vi "Teststand Edit STP Sent Command.vi"(8 "error in":errorcluster, 10 "STP Set Profile Data in":T1={"ECU CAN Port"="CAN1", "CMD"=133, "CAN Write Data"=[], "+veResponseCode"=160} {"+veResponseCode" format="%.0x"; "CMD" items=["TSW_VERSION(130)"=130, "WAIT_EVENT(132)"=132, "SEQUENCER(133)"=133, "TSW_RESET(150)"=150, "CONFIG_ECU(151)"=151, "TEST_CORE (152)"=152, "TEST_WATCHDOG (153)"=153, "TEST_MONITORING (154)"=154, "READ_MEMORY (162)"=162, "WRITE_ERASE_MEMORY (164)"=164, "COMM_EXTERNAL (190)"=190, "COMM_INTERNAL (195)"=195, "GET_ANALOG_INPUT (210)"=210, "GET_DIGITAL_INPUT (211)"=211, "GET_FREQUENCY_INPUT (212)"=212, "TEST_INPUT_STRUCTURE (214)"=214, "GENERATE_OUTPUT_SIGNAL (220)"=220, "GENERATE_SYNCHRONIZED_OUTPUT_SIGNALS (221)"=221, "eDCU_Specific (250)"=250]; "CAN Write Data" format="%.0x"}, 11 "Sequence Context In":refnum<k7>) -> (0 "error out":errorcluster, 3 "STP Profile Data Out":T1={"ECU CAN Port"="CAN1", "CMD"=133, "CAN Write Data"=[], "+veResponseCode"=160} {"+veResponseCode" format="%.0x"; "CMD" items=["TSW_VERSION(130)"=130, "WAIT_EVENT(132)"=132, "SEQUENCER(133)"=133, "TSW_RESET(150)"=150, "CONFIG_ECU(151)"=151, "TEST_CORE (152)"=152, "TEST_WATCHDOG (153)"=153, "TEST_MONITORING (154)"=154, "READ_MEMORY (162)"=162, "WRITE_ERASE_MEMORY (164)"=164, "COMM_EXTERNAL (190)"=190, "COMM_INTERNAL (195)"=195, "GET_ANALOG_INPUT (210)"=210, "GET_DIGITAL_INPUT (211)"=211, "GET_FREQUENCY_INPUT (212)"=212, "TEST_INPUT_STRUCTURE (214)"=214, "GENERATE_OUTPUT_SIGNAL (220)"=220, "GENERATE_SYNCHRONIZED_OUTPUT_SIGNALS (221)"=221, "eDCU_Specific (250)"=250]; "CAN Write Data" format="%.0x"})   [LabVIEW 2023, in "LTT_TeststandSteptypes.lvlib"]
uses:
  LTT_TeststandSteptypes.lvlib
  Control/STP Sent Command.ctl
  HardwareAbstractionLayer_LVOOP/CAN/CAN Application Protocols/STP Protocol_class/Ctrls/STP CMD.ctl
  <vilib>/addons/TestStand/_TSUtility.llb/TestStand - Start Modal Dialog (Sequence Context).vi
  <vilib>/addons/TestStand/_TSUtility.llb/TestStand - End Modal Dialog (Sequence Context).vi
  HardwareAbstractionLayer_LVOOP/Database/Database.lvclass
  HardwareAbstractionLayer_LVOOP/Database/SQL Public VI/Control/DB Options.ctl
  HardwareAbstractionLayer_LVOOP/CAN/CAN Application Protocols/STP Protocol_class/STP Protocol.lvclass
panel:
  in  "Close":bool
  in  "OK":bool
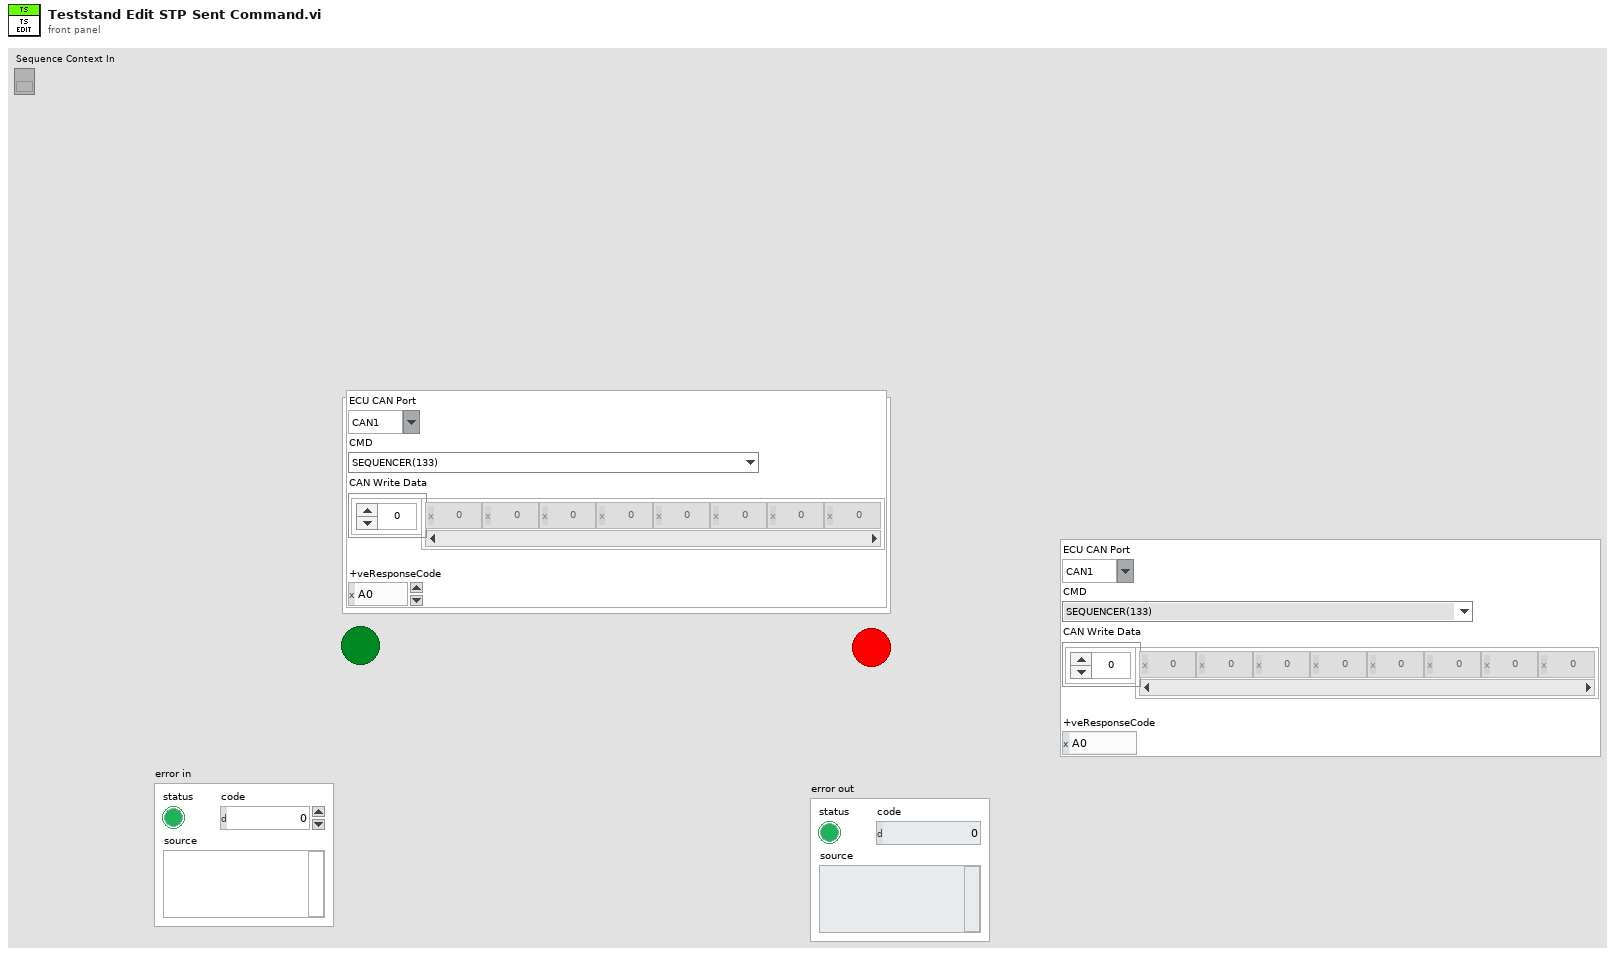
[diagram p1: front panel]
types:
  T1 = typedef "LTT_TeststandSteptypes.lvlib/STP Sent Command.ctl" = cluster{"ECU CAN Port":string, "CMD":T2, "CAN Write Data":u8[], "+veResponseCode":u8}
  T2 = typedef "HardwareAbstractionLayer_LVOOP.lvlib/CAN Application Protocols Lib.lvlib/STP Protocol.lvclass/STP CMD.ctl" = u8
  T3 = typedef "HardwareAbstractionLayer_LVOOP.lvlib/Database.lvclass/DB Options.ctl" = enum16{"Init", "Select Data", "Insert Data", "Update Data", "Delete Data", "Execute Query", "Create Schema", "Create Table", "List Tables", "List Columns", "Close"}
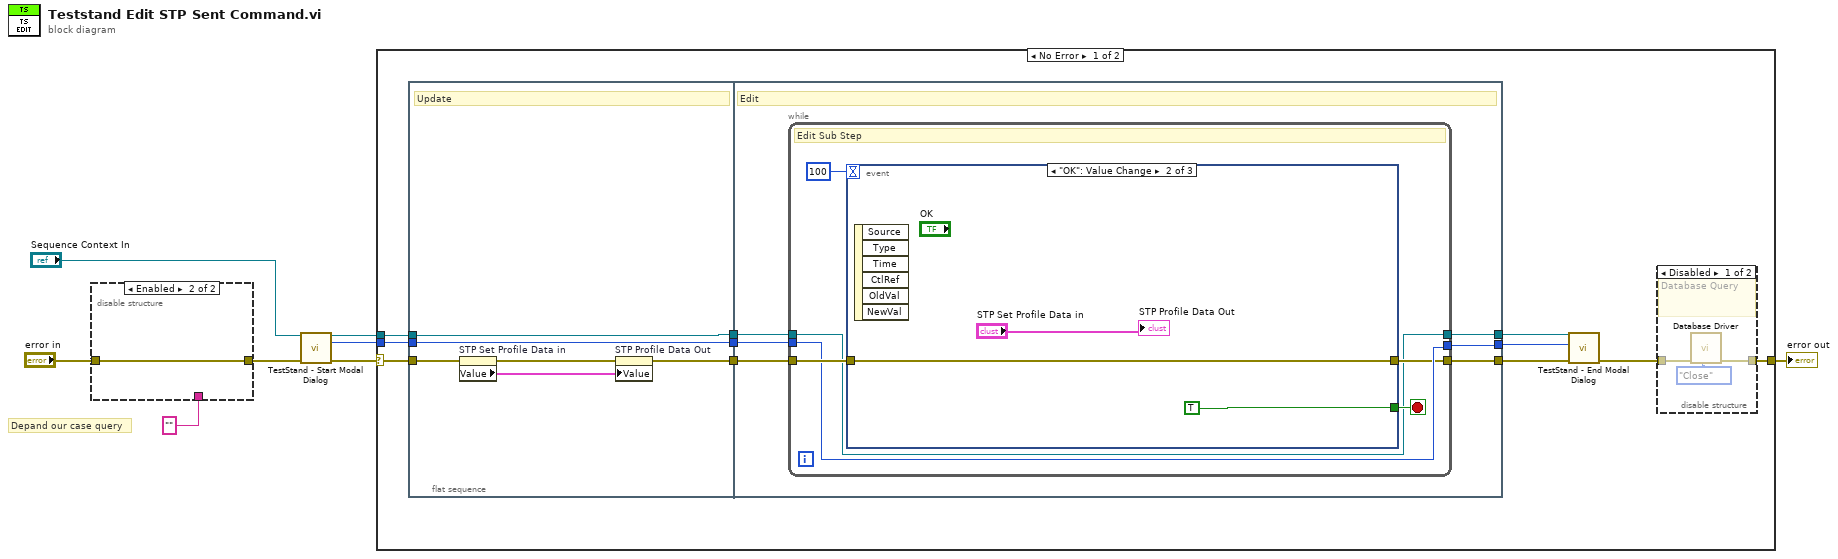
[diagram p0: block diagram]
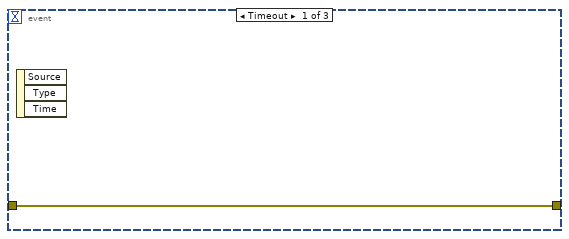
[diagram p3: hidden frame]
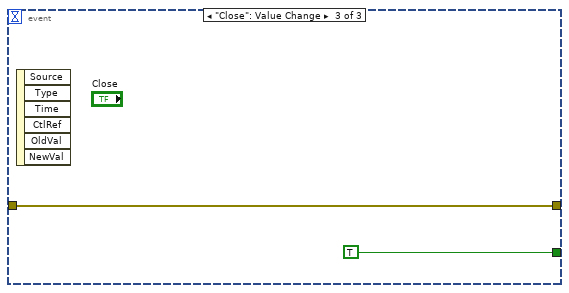
[diagram p4: hidden frame]
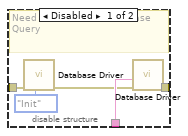
[diagram p6: hidden frame]
diagram:
  # "Depand our case query"
  n1 = disable-structure shown="Enabled" {
    disable-tunnel: "error in" -> [w13 w14]
    disable-tunnel: [w12 w14] -> w3
    disable-tunnel: "" ("SQL query") -> [w11 _]
    frame Disabled {
      # "Need to Enable for Database Query"
      n2 = call "Database Driver.vi"("Options"=DB_Options."Init", "error in"=w13) -> ("error out"=w10:errorcluster)  [unwired: 6 in, 3 out]
      n3 = call "Database Driver.vi"("error in"=w10, "SQL query"=w11) -> ("error out"=w12:errorcluster)  [unwired: 6 in, 3 out]
    }
    frame Enabled {
    }
  }
  n4 = call-poly <vilib>:"TestStand - Start Modal Dialog.vi"("Sequence Context In"="Sequence Context In", "error in (no error)"=w3) -> ("Sequence Context Out"=w5:refnum<k7>, "Modal ID"=w4:i32, "error out"=w6:errorcluster)  [unwired: 9 in, 2 out]
  n5 = case shown="No Error" w6 {
    selector: w6 -> [w22 w53]
    tunnel: w5 -> [w19 _]
    tunnel: w4 -> [w18 _]
    tunnel: [w16 w53] -> w1
    frame No Error {
      n6 = flat-sequence {
        tunnel: w22 -> [w31]
        tunnel: [w32] -> w25
        tunnel: w19 -> [w34]
        tunnel: w18 -> [w33]
        tunnel: [w34] -> w24
        tunnel: [w33] -> w23
        tunnel: w25 -> [w38]
        tunnel: [w36] -> w21
        tunnel: w24 -> [w40]
        tunnel: w23 -> [w39]
        tunnel: [w37] -> w17
        tunnel: [w35] -> w15
        frame #0 {
          # "Update"
          n7 = property on="STP Set Profile Data in" class="Clust (strict)"(error in=w31) -> (error out=w29:errorcluster, "Value"=w30:T1)  [unwired: 1 in, 1 out]
          n8 = property on="STP Profile Data Out" class="Clust (strict)"(error in=w29, "Value"=w30) -> (error out=w32:errorcluster)  [unwired: 1 in, 1 out]
        }
        frame #1 {
          # "Edit"
          n9 = while {
            tunnel: w40 -> [w41]
            tunnel: w39 -> [w43]
            tunnel: w38 -> [w44]
            tunnel: [w43] -> w37
            tunnel: [w42] -> w36
            tunnel: [w41] -> w35
            stop <- w45 stop-if-true
            # "Edit Sub Step"
            n10 = event shown="[1] \"OK\": Value Change" {
              selector: _ -> [_ _ _]
              dyn-events: _ -> [_ _ _]
              timeout: 100 -> [_ _ _]
              tunnel: [_ TRUE TRUE] -> w45
              tunnel: w44 -> [w47 w49 w51]
              tunnel: [w47 w49 w51] -> w42
              event Timeout {
                n11 = event-data() -> ()  [unwired: 1 in, 3 out]
              }
              event "OK": Value Change {
                n12 = event-data() -> ()  [unwired: 1 in, 6 out]
                "STP Profile Data Out" <- "STP Set Profile Data in"
              }
              event "Close": Value Change {
                n13 = event-data() -> ()  [unwired: 1 in, 6 out]
              }
            }
          }
        }
      }
      n14 = call-poly <vilib>:"TestStand - End Modal Dialog.vi"("Sequence Context In"=w15, "Modal ID"=w17, "error in (no error)"=w21) -> ("error out"=w20:errorcluster)  [unwired: 12 in]
      n15 = disable-structure shown="Disabled" {
        disable-tunnel: w20 -> [w28 _]
        disable-tunnel: [w27 _] -> w16
        frame Disabled {
          # "Need to Enable for Database Query"
          n16 = call "Database Driver.vi"("Options"=DB_Options."Close", "error in"=w28) -> ("error out"=w27:errorcluster)  [unwired: 6 in, 3 out]
        }
        frame Enabled {
        }
      }
    }
    frame Error {
    }
  }
  "error out" <- w1
